vi "Write Local Resource.vi"(8 "error in (no error)":errorcluster, 10 "Local Resource":refnum<visa-resource-name>, 11 "69X_79X In":refnum<class "7976A.lvclass">) -> (0 "error out":errorcluster, 3 "69X_79X Out":refnum<class "7976A.lvclass">)   [LabVIEW 2019, in "7976A.lvlib" / "7976A.lvclass"]
uses:
  Library/7976A.lvclass
  Library/7976A.lvclass/7976A.ctl
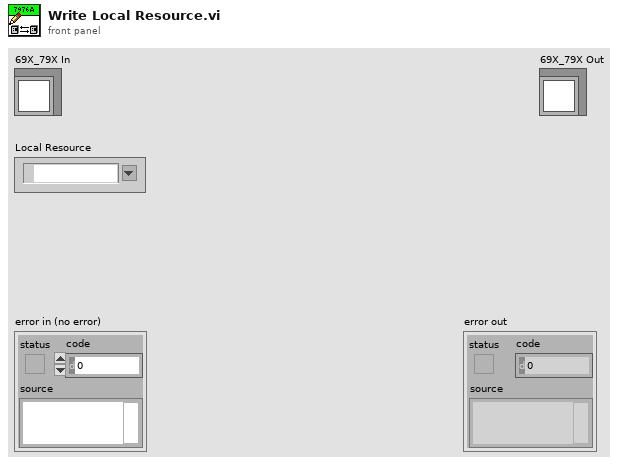
[diagram p1: front panel]
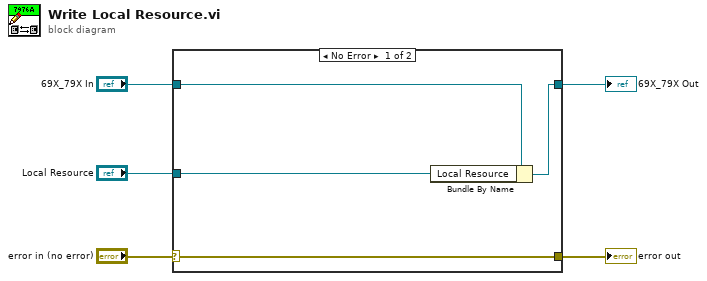
[diagram p0: block diagram]
diagram:
  n1 = case shown="No Error" "error in (no error)" {
    selector: "error in (no error)" -> [w9 w10]
    tunnel: [w9 w10] -> w1
    tunnel: [w7 w11] -> w4
    tunnel: "69X_79X In" -> [w8 w11]
    tunnel: "Local Resource" -> [w6 _]
    frame No Error {
      n2 = Bundle By Name(cluster=w8, "Local Resource"=w6) -> (w7:refnum<class "7976A.lvclass">)
    }
    frame Error {
    }
  }
  "69X_79X Out" <- w4
  "error out" <- w1
